vi "Receive - UDP (SAP).vi"() -> ()   [LabVIEW 2020]
uses:
  _controls/comm_verification_rx.ctl
  _controls/sap_config_rx.ctl
  _polimorphicInstances/session/Fdx Create Session (Rx-VL-Oriented).vi
  bsp/AFDX_Receive/Fdx Create Rx VL.vi
  _polimorphicInstances/udpPort/Fdx Create Udp Port (RX-SAP).vi
  _polimorphicInstances/control/Fdx Start (Rx).vi
  _polimorphicInstances/control/Fdx Stop (Rx).vi
  _polimorphicInstances/session/Fdx Close Session (Port).vi
  AIM664LV.lvlib
panel:
  out "MsgErrorCount":u32
  in  "Period mS":u32=200
  out "MsgRead":u32
  out "Data":u8[][](array[numeric])=[[1, 2, 3, 4, 0, 0, 0, 0, 0, 0, 0, 0, 0, 0, 0, 0, 0, 0, 0, 0, 0, 0, 0, 0, 0, 0, 0, 0, 0, 0, 0, 0, 0, 0, 0, 0, 0, 0, 0, 0, 0, 0, 0, 0, 0, 0, 0, 0, 0, 0, 0, 0, 0, 0, 0, 0, 0, 0, 0, 0, 0, 0, 0, 0, 0, 0, 0, 0, 0, 0, 0, 0, 0, 0, 0, 0, 0, 0, 0, 0, 0, 0, 0, 0, 0, 0, 0, 0, 0, 0, 0, 0, 0, 0, 0, 0, 0, 0, 0, 0]] format="%.0x"
  in  "Messages to Read (1)":u32=1
  in  "SapPort Config":T1={"UdpDstPort"=12345, "UdpNumBufMessages"=0, "UdpMaxMessageSize"=0}
  in  "VL Config":T2={"VlId"=60, "VLRange"=2, "VerificationMode"=0, "Bag"=0, "Jitter"=0, "MaxFrameLength"=0, "MaxSkew"=0, "VLBufSize"=32768, "FilterMode"=0, "FilterPosition"=0, "Padding"=0, "FilterMask"=0, "FilterData"=0, "MinFrameLength"=0} {"FilterMode" items=["FDX_RX_VL_FLT_DIS", "FDX_RX_VL_FLT_ENA ", "FDX_RX_VL_FLT_ENA_INV"]; "MaxFrameLength" format="%.0x"; "VerificationMode" items=["FDX_RX_VL_CHECK_ENA_DEFAULT"=65535, "FDX_RX_VL_CHECK_REDMAM"=16, "DX_RX_VL_CHECK_TRAFIC"=8, "FDX_RX_VL_CHECK_FRAMESIZE"=4, "FDX_RX_VL_CHECK_SNINTEG"=2, "FDX_RX_VL_CHECK_INVPAC"=1, "FDX_RX_VL_CHECK_DISA"=0]}
  out "PortInitOut":T3={"PortConfig"=0, "PortUsed"=1, "GlobalMemFree"=0, "SharedMemFree"=0} {"PortConfig" items=["FDX_SINGLE", "FDX_REDUNDANT"]}
  in  "Port":u32
  in  "Board":u32
  out "error out":errorcluster
  in  "stop":bool
  out "current time":timestamp
  # "ARINC 664 - Receiving through UDP with a Service Access Point (SAP)"
  # "Overview: Setup the board to transmit package as raw frames.\nRequirement: One AIM ARINC-664 board with installed AIM ARINC 664 BSP.\nRestrictions: None.\nInstruction:\n1. Select the Board ID (0 if you have only one board in your system) and the port number. If you want to validate between two ports in one device, you can use tx board and Rx Board\n2. Run the VI.\n3. See the result in Current IRIG Time"
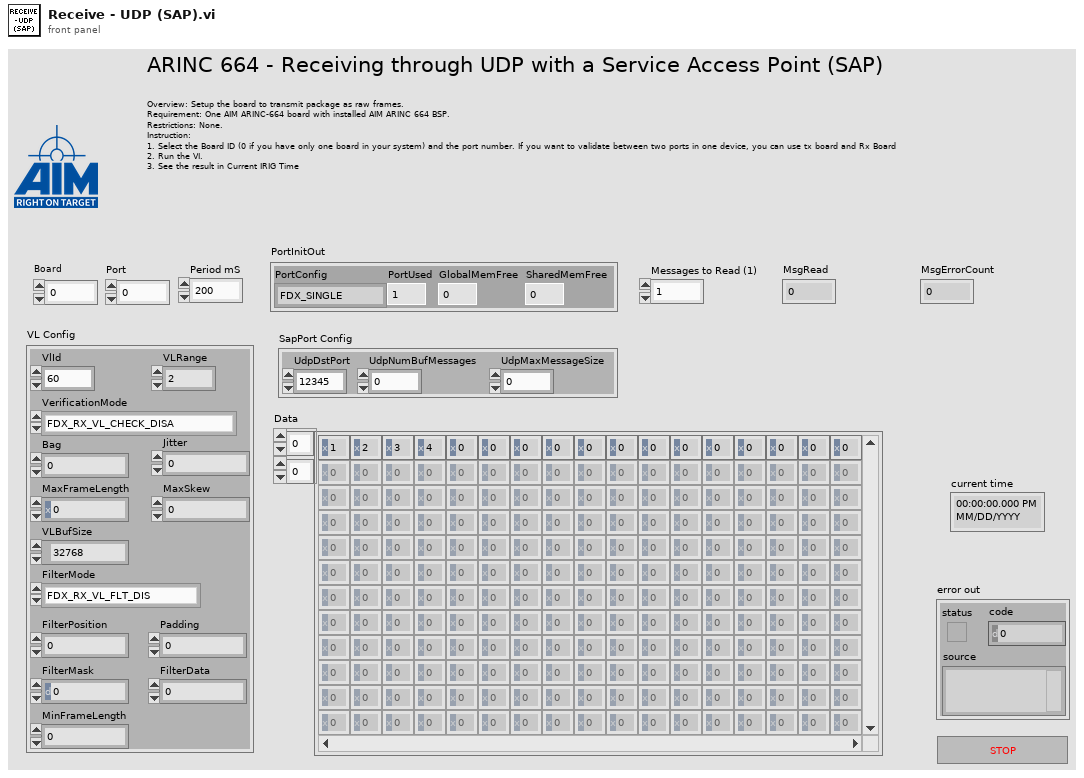
[diagram p1: front panel]
types:
  T1 = typedef "AIM664LV.lvlib/sap_config_rx.ctl" = cluster{"UdpDstPort":u16, "UdpNumBufMessages":u32, "UdpMaxMessageSize":u32}
  T2 = typedef "AIM664LV.lvlib/comm_verification_rx.ctl" = cluster{"VlId":u16, "VLRange":u32, "VerificationMode":u32, "Bag":u32, "Jitter":u32, "MaxFrameLength":u32, "MaxSkew":u32, "VLBufSize":u32, "FilterMode":u32, "FilterPosition":u32, "Padding":u32, "FilterMask":u32, "FilterData":u32, "MinFrameLength":u32}
  T3 = cluster{"PortConfig":u32, "PortUsed":u32, "GlobalMemFree":u32, "SharedMemFree":u32}
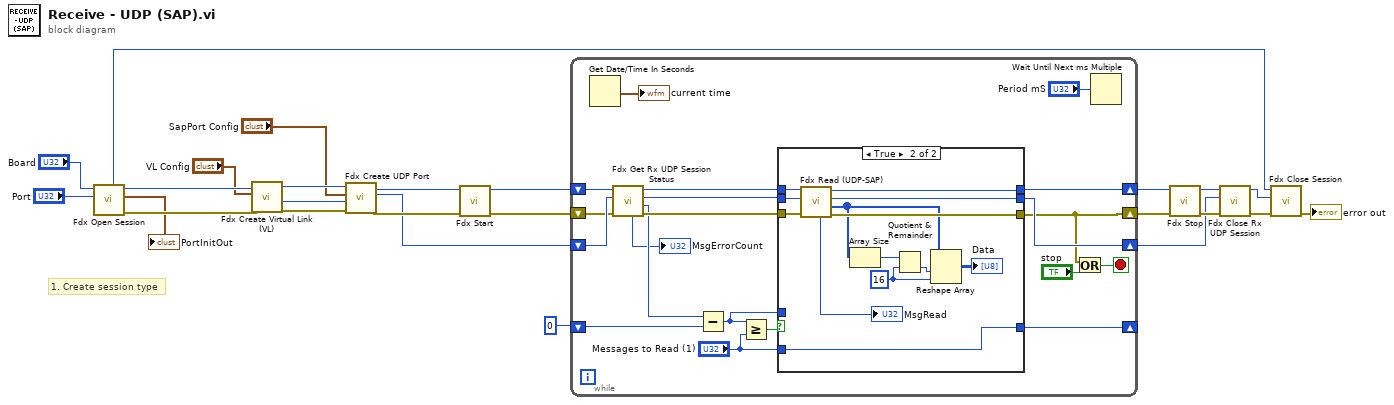
[diagram p0: block diagram]
diagram:
  # "1. Create session type"
  n1 = call-poly "Fdx Open Session.vi"("port"="Port", "board"="Board") -> ("error out"=w24:errorcluster, "PortInitOut"=→"PortInitOut":T3, "InstrumentHandle_port out"=w25:u32, "InstrumentHandle_board out"=w3:u32)  [unwired: 4 in, 2 out]
  n2 = call-poly "Fdx Create Virtual Link (VL).vi"("error in (no error)"=w24, "VL Config"="VL Config", "InstrumentHandle_port in"=w25) -> ("error out"=w22:errorcluster, "VlId"=w7:u16, "InstrumentHandle_port out"=w23:u32)  [unwired: 6 in]
  n3 = call-poly "Fdx Create UDP Port.vi"("error in (no error)"=w22, "VlId"=w7, "SapPort Config"="SapPort Config", "port handle in"=w23) -> ("error out"=w20:errorcluster, "sapPort handle out"=w17:u32, "port handle out"=w21:u32)  [unwired: 4 in, 1 out]
  n4 = call-poly "Fdx Start.vi"("error in (no error)"=w20, "InstrumentHandle_port in"=w21) -> ("error out"=w2:errorcluster, "InstrumentHandle_port out"=w19:u32)  [unwired: 8 in]
  n5 = while {
    shift-right: [w35] -> w18
    shift-left: w19 -> [w36]
    shift-right: [w32] -> w6
    shift-left: w17 -> [w34]
    shift-right: [w38] -> _
    shift-left: u32 0 ("MsgCount") -> [w44]
    shift-right: [w28] -> w1
    shift-left: w2 -> [w31]
    stop <- w27 stop-if-true
    n6 = Get Date/Time In Seconds() -> (seconds since 1Jan1904=→"current time":timestamp)
    n7 = call "Fdx Get Rx UDP Session Status.vi"("error in (no error)"=w31, "UdpHandle in"=w34, "InstrumentHandle_port in"=w36) -> ("error out"=w43:errorcluster, "MsgCount"=w37:u32, "UdpHandle out"=w33:u32, "InstrumentHandle_port out"=w42:u32, "MsgErrorCount"=→"MsgErrorCount":u32)  [unwired: 4 in]
    n8 = Subtract(x=w37, y=w44) -> (x-y=w39:u32)
    n9 = Greater Or Equal?(x=w39, y="Messages to Read (1)") -> (x >= y?=w41:bool)
    n10 = case shown="True" w41 {
      tunnel: w43 -> [w47 w60]
      tunnel: w42 -> [w49 w61]
      tunnel: "Messages to Read (1)" -> [_ w62]
      tunnel: [w49 w59] -> w35
      tunnel: w39 -> [w48 _]
      tunnel: [w48 w62] -> w38
      tunnel: [w47 w58] -> w28
      tunnel: w33 -> [w46 w57]
      tunnel: [w46 w56] -> w32
      frame False {
      }
      frame True {
        w52 = 16 ("dimension size")
        n11 = call "Fdx Read (UDP-SAP).vi"("error in"=w60, "UdpHandle in"=w57, "InstrumentHandle_port in"=w61) -> ("error out"=w58:errorcluster, "Data"=w51:u8[], "UdpHandle out"=w56:u32, "InstrumentHandle_port out"=w59:u32, "MsgRead"=→"MsgRead":u32)  [unwired: 4 in]
        n12 = Array Size(array=w51) -> (size(s)=w53:i32)
        n13 = Quotient & Remainder(x=w53, y=w52) -> (floor(x/y)=w54:i32)  [unwired: 1 out]
        n14 = Reshape Array(w51, w54, w52) -> (→"Data":u8[][])
      }
    }
    n15 = Or(x=w28, y="stop") -> (x .or. y?=w27:bool)
    n16 = Wait Until Next ms Multiple(millisecond multiple="Period mS") -> ()  [unwired: 1 out]
  }
  n17 = call-poly "Fdx Stop.vi"("error in (no error)"=w1, "InstrumentHandle_port in"=w18) -> ("error out"=w16:errorcluster, "InstrumentHandle_port out"=w5:u32)  [unwired: 8 in]
  n18 = call "Fdx Close Rx UDP Session.vi"("error in (no error)"=w16, "UdpHandle in"=w6, "InstrumentHandle_port in"=w5) -> ("error out"=w15:errorcluster, "InstrumentHandle_port out"=w4:u32)  [unwired: 7 in]
  n19 = call-poly "Fdx Close Session.vi"("error in"=w15, "InstrumentHandle_port in"=w4, "InstrumentHandle_board in"=w3) -> ("error out"=→"error out":errorcluster)  [unwired: 8 in]
